vi "infinete run.vi"() -> ()   [LabVIEW 2010]
uses:
  <vilib>/NXT/Subs/MotorOutput.ctl
  <vilib>/NXT/Dual Mode Library/Motors/MotorOn.vi
panel:
  in  "stop":bool
  in  "Output Port (All Ports)":T1=3 items=["Port A", "Port B", "Port C", "All Ports"]
  in  "Power (75)":i32=75
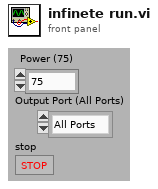
[diagram p1: front panel]
types:
  T1 = typedef "MotorOutput.ctl" = u8
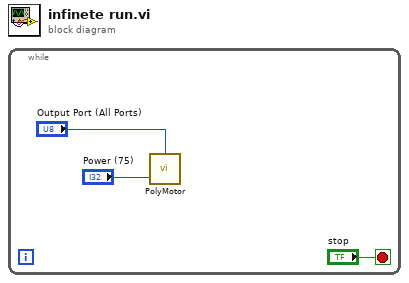
[diagram p0: block diagram]
diagram:
  n1 = while {
    stop <- "stop" stop-if-true
    n2 = call-poly <vilib>:"PolyMotor.vi"("Power (75)"="Power (75)", "Output Port (All Ports)"="Output Port (All Ports)") -> ()  [unwired: 2 in, 1 out]
  }
